vi "Initialize.vi"(8 "error in (no error)":errorcluster) -> (0 "error out":errorcluster, 1 "Exit Event":refnum<user-event>, 2 "Queue":refnum<queue>, 3 "Event Registration Refnum":refnum<event-registration>)   [LabVIEW 2020, in "Code Cleanup.lvlib" / "FaKI State Machine.lvlib"]
doc: "Initializes and registers for the \"Exit\" user event. Initializes the queue and enqueues the \"Macro: Initialize\" state.\n\nThis VI is inlined."
uses:
  FaKI State Machine.lvlib
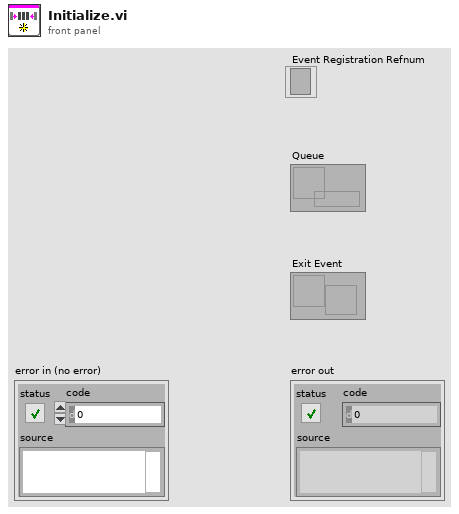
[diagram p1: front panel]
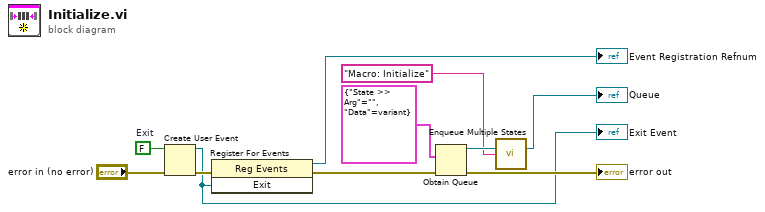
[diagram p0: block diagram]
diagram:
  w8 = FALSE  # Exit
  n1 = Create User Event(user event datatype=w8, error in="error in (no error)") -> (user event=w2:refnum<user-event>, error out=w9:errorcluster)
  "Exit Event" <- w2
  n2 = register-events(error in=w9, w2) -> (reference out=→"Event Registration Refnum":refnum<event-registration>, error out=w7:errorcluster)  [unwired: 1 in]
  n3 = Obtain Queue(element data type=cluster{"State >> Arg":string, "Data":variant} {"State >> Arg"="", "Data"=variant}, error in (no error)=w7) -> (queue out=w10:refnum<queue>, error out=→"error out":errorcluster)  [unwired: 3 in, 1 out]
  n4 = call "Enqueue Multiple States.vi"("queue in"=w10, "State(s) at Back"="Macro: Initialize") -> ("queue out"=→"Queue":refnum<queue>)  [unwired: 13 in]
